vi "UpdateTarget Time.vi"(8 "error in":errorcluster) -> (0 "error out":errorcluster)   [LabVIEW 2012]
uses:
  <vilib>/nisyscfg/nisyscfg.lvlib
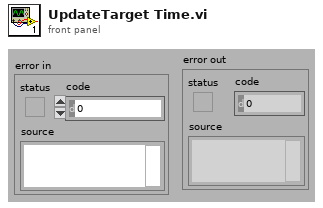
[diagram p1: front panel]
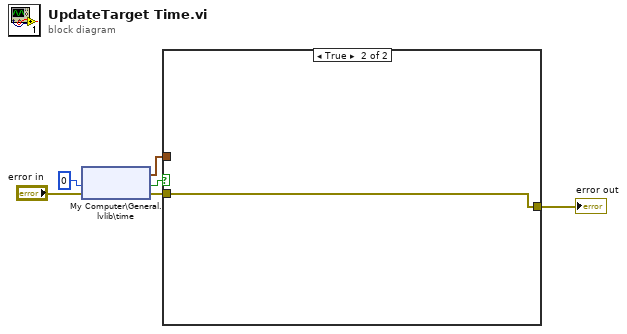
[diagram p0: block diagram]
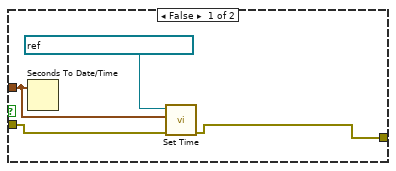
[diagram p2: hidden frame]
diagram:
  n1 = shared-variable "My Computer\\General.lvlib\\time"(error in="error in", 0 ("ms timeout (0)")) -> (w2:timestamp, error out=w5:errorcluster, w3:bool)
  n2 = case shown="True" w3 {
    tunnel: w5 -> [w9 w11]
    tunnel: w2 -> [w10 _]
    tunnel: [w7 w11] -> w1
    frame False {
      n3 = Seconds To Date/Time(time stamp (now)=w10) -> ()  [unwired: 1 in, 1 out]
      n4 = call <vilib>:"Set Time.vi"("error in (no error)"=w9, "time"=w10, "session in (localhost)"=refnum<k21> "CRDS-PAS (10.172.240.107)") -> ("error out"=w7:errorcluster)  [unwired: 5 in, 3 out]
    }
    frame True {
    }
  }
  "error out" <- w1
